vi "Error Dequeue.vi"(8 "error in":errorcluster, 10 "Error Queue in":refnum<queue>) -> (0 "error out":errorcluster, 3 "Error Message":refnum<class "Error.lvclass">)   [LabVIEW 2017, in "TSC Error.lvlib"]
doc: "This VI will handle dequeing messages from the Error Queue.\n\nInputs:\n-Error Queue in [Queue reference] - the Error Queue\n-error in\n\nOutputs:\n-Error Message [obj] - the dynamic dispatch output class message\n-error out\n________________________________________________________________________________\n<b>Code Developed By:</b>\nDaniel Coons\nTechnology Service Corporation\n1983 S Liberty Drive\nBloomington, IN 47403\nPhone: 812 558-7100\ndaniel.coons@tsc.com\nwww.tsc.com\n\n<b>Date Created:</b> 11 AUG 2014\n<b>Date Updated:</b>"
uses:
  TSC Error.lvlib
  _Messages/Error/Error.lvclass
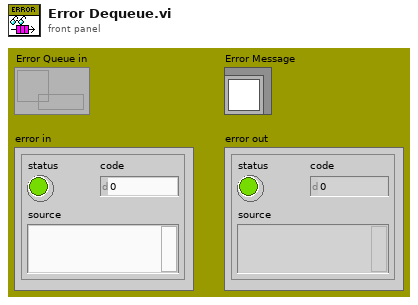
[diagram p1: front panel]
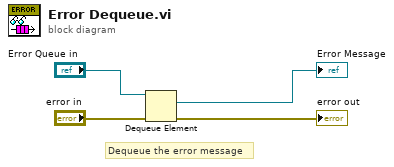
[diagram p0: block diagram]
diagram:
  # "Dequeue the error message"
  n1 = Dequeue Element(queue="Error Queue in", error in (no error)="error in") -> (element=→"Error Message":refnum<class "Error.lvclass">, error out=→"error out":errorcluster)  [unwired: 1 in, 2 out]
